vi "WCA_SET_CLNA.vi"(0 "Cartridge Band":u32=10, 1 "Slave Node in":cluster{"Address":i16, "Serial Number":i8[]}={"Address"=19, "Serial Number"=[16, 71, 55, 76, 1, 8, 0, -15]} {"Serial Number" format="%.0x"; "Address" format="%.0x"}, 2 "ObjHandle in":u32, 5 "POL":u32, 7 "sb":u32=1, 9 "CLNA_SET":T1 {"SET POL0 LNA1 STAGE3 DRAIN C" min=0 max=20 step=0.01 format="%.2f"; "SET POL0 LNA1 STAGE3 DRAIN V" min=0 max=3 step=0.01 format="%.2f"; "SET POL0 LNA1 STAGE2 DRAIN C" min=0 max=20 step=0.01 format="%.2f"; "SET POL0 LNA1 STAGE2 DRAIN V" min=0 max=3 step=0.01 format="%.2f"; "SET POL0 LNA1 STAGE1 DRAIN C" min=0 max=20 step=0.01 format="%.2f"; "SET POL0 LNA1 STAGE1 DRAIN V" min=0 max=3 step=0.01 format="%.2f"; "CLNA State" items=["Disabled", "Enabled"]}, 11 "error in (no error)":errorcluster) -> (4 "ObjHandle out":u32=92930112, 15 "error out":errorcluster)   [LabVIEW 2017]
uses:
  WCA_Global.vi
  <vilib>/express/express arith-compare/Formula/XNode/ExpressFormulaBlockNode.xnode
panel:
  # "Node Address"
  # "Serial Number"
  # "Vd [V]"
  # "Id [mA]"
  # "Stage 1"
  # "Stage 2"
  # "Stage 3"
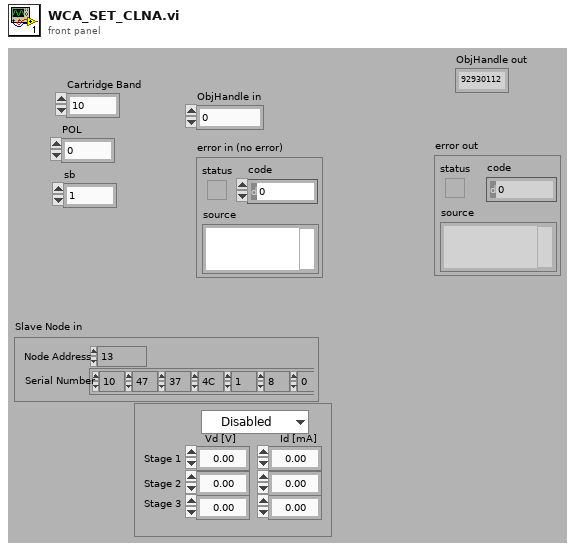
[diagram p1: front panel]
types:
  T1 = cluster{"CLNA State":u8, "SET POL0 LNA1 STAGE1 DRAIN V":sgl, "SET POL0 LNA1 STAGE1 DRAIN C":sgl, "SET POL0 LNA1 STAGE2 DRAIN V":sgl, "SET POL0 LNA1 STAGE2 DRAIN C":sgl, "SET POL0 LNA1 STAGE3 DRAIN V":sgl, "SET POL0 LNA1 STAGE3 DRAIN C":sgl}
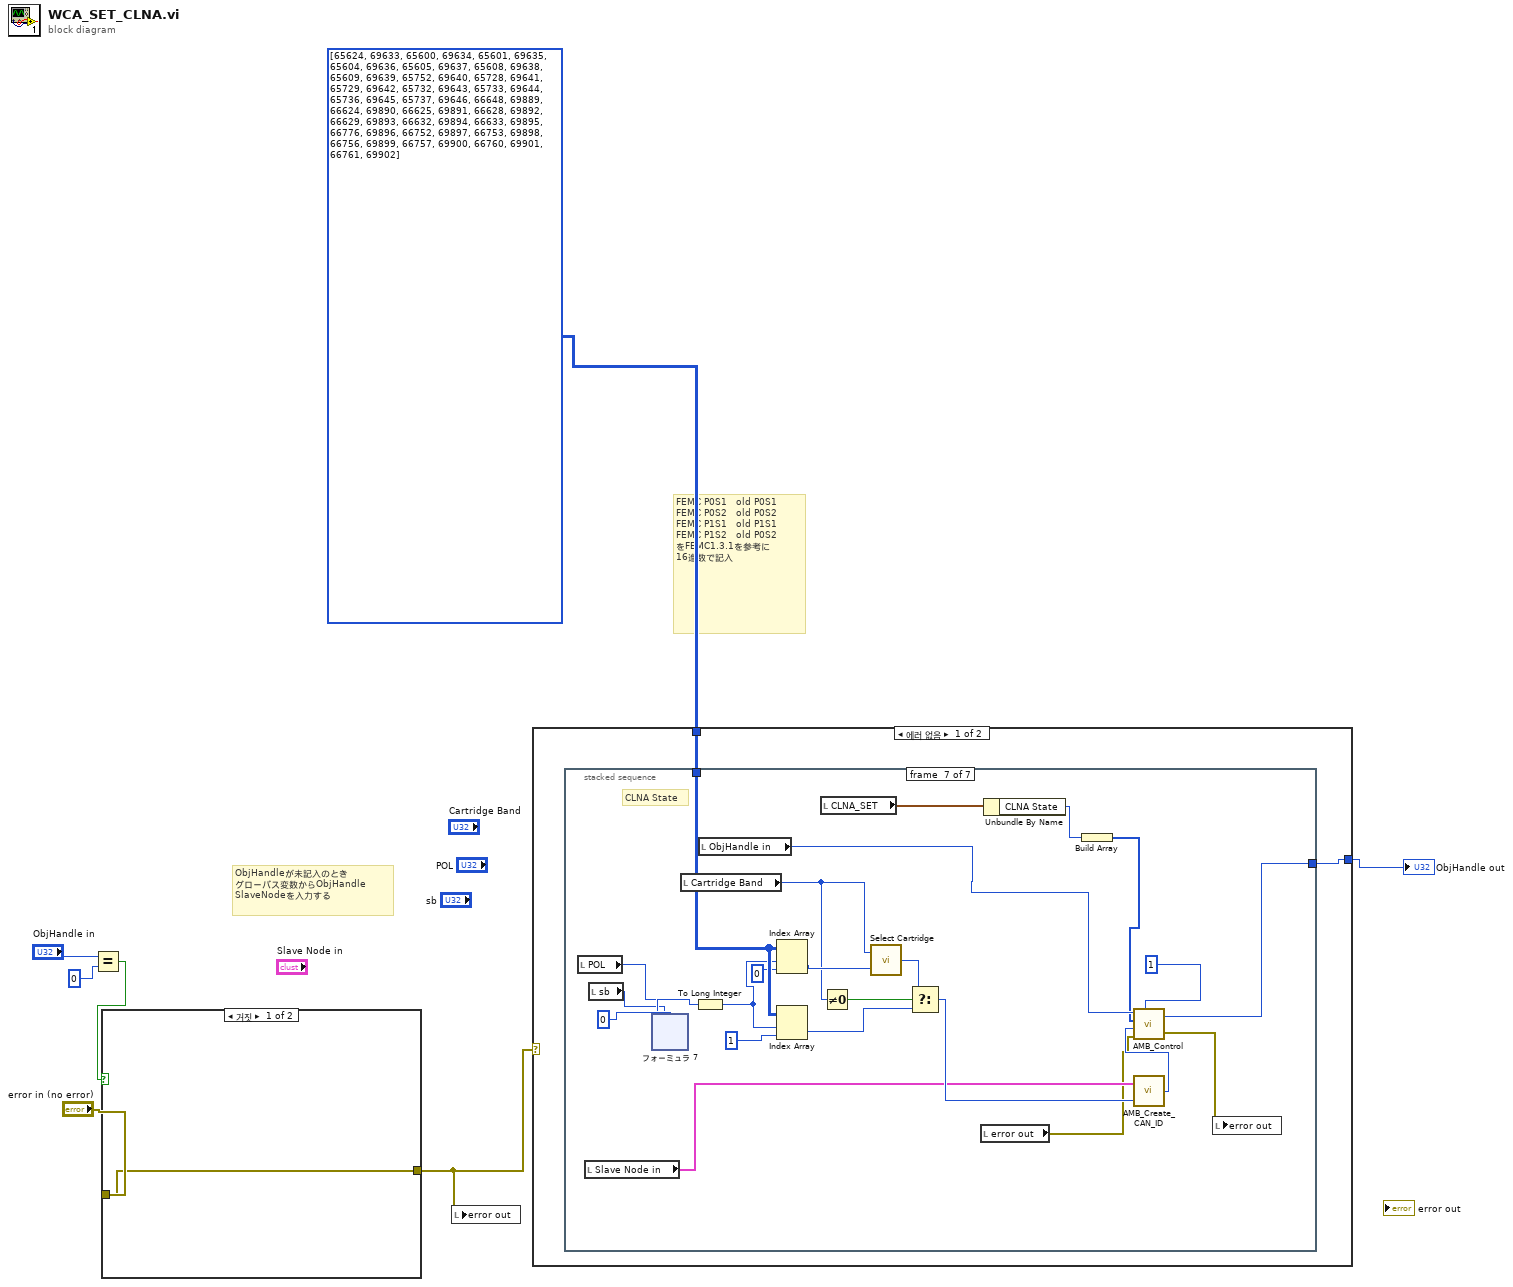
[diagram p0: block diagram]
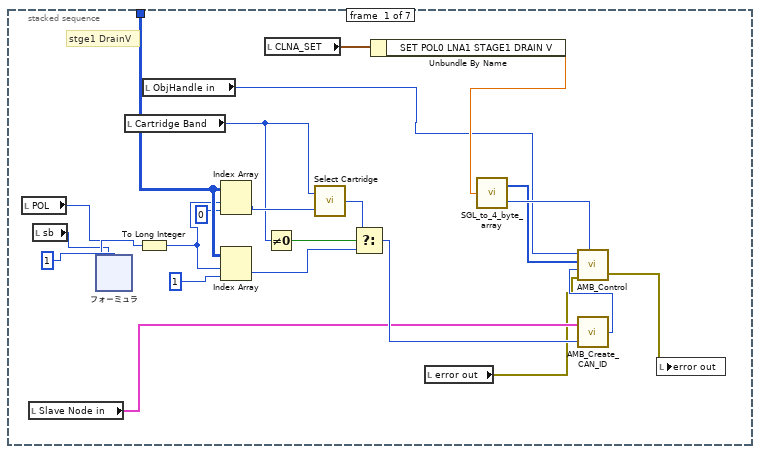
[diagram p2: hidden frame]
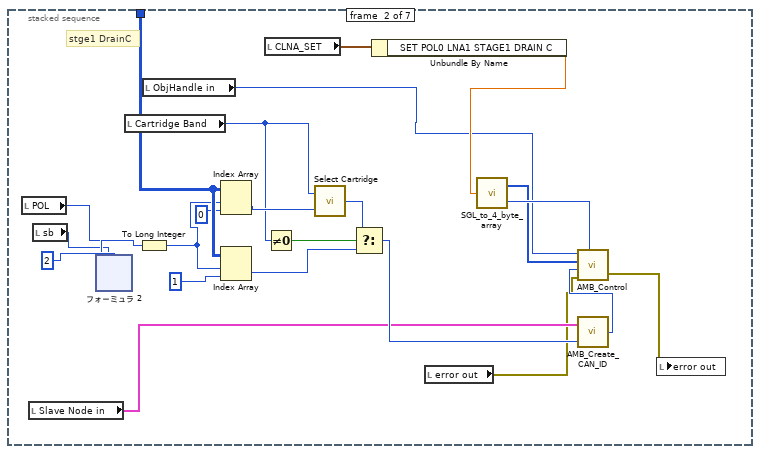
[diagram p3: hidden frame]
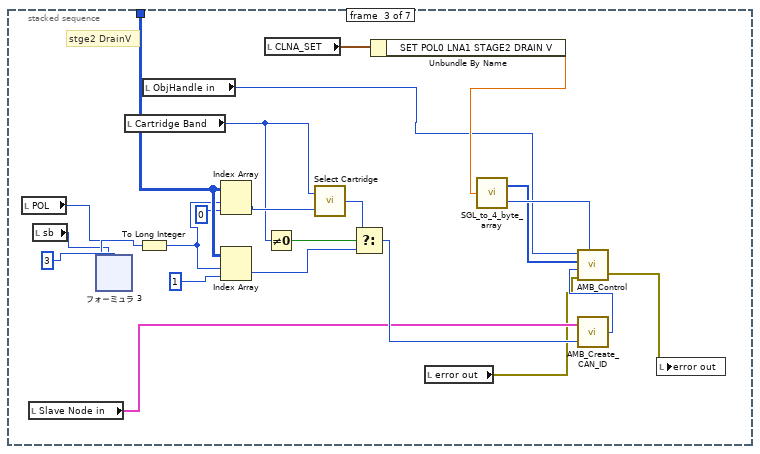
[diagram p4: hidden frame]
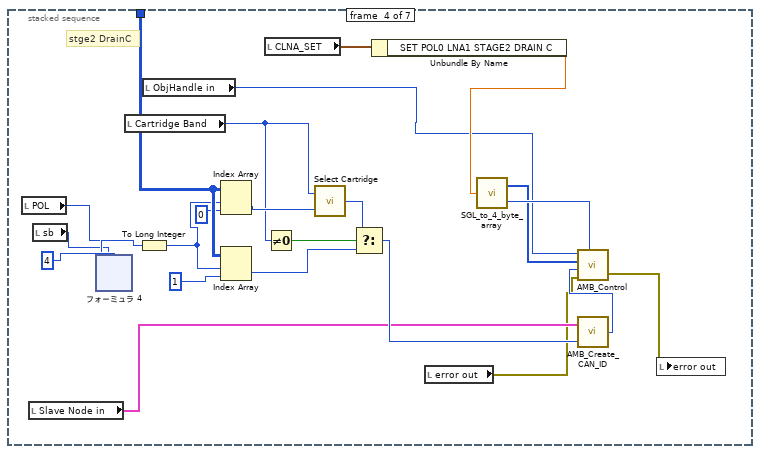
[diagram p5: hidden frame]
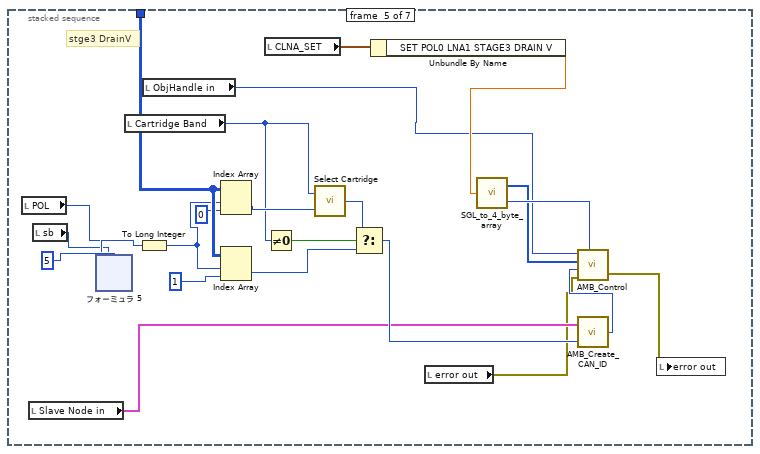
[diagram p6: hidden frame]
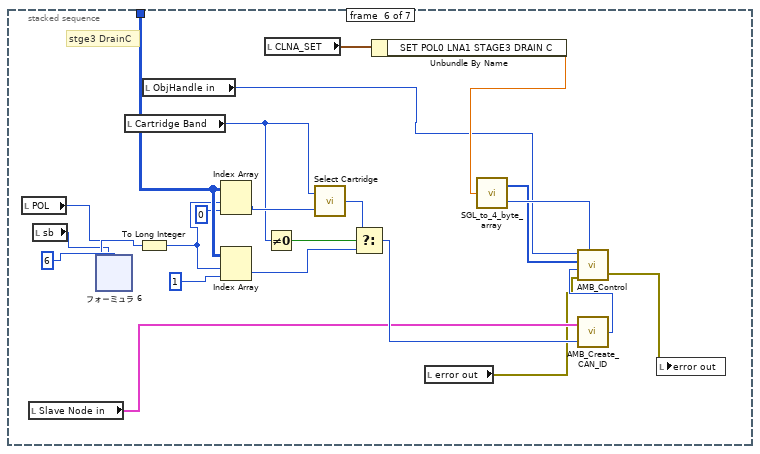
[diagram p7: hidden frame]
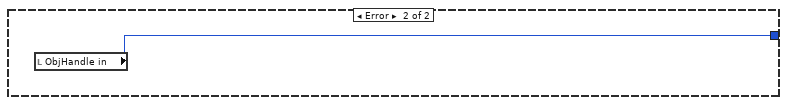
[diagram p8: hidden frame]
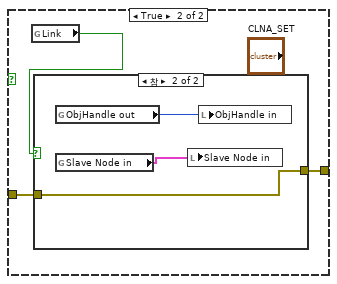
[diagram p9: hidden frame]
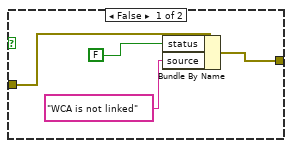
[diagram p10: hidden frame]
diagram:
  # "ObjHandleが未記入のとき\nグローバス変数からObjHandle\nSlaveNodeを入力する"
  # "FEMC P0S1   old P0S1\nFEMC P0S2   old P0S2\nFEMC P1S1   old P1S1\nFEMC P1S2   old P0S2\nをFEMC1.3.1を参考に\n16進数で記入"
  n1 = Equal?(x="ObjHandle in", y=0) -> (x = y?=w5:bool)
  n2 = case shown="거짓" w5 {
    tunnel: "error in (no error)" -> [w8 w11]
    tunnel: [w8 w10] -> w3
    frame False {
    }
    frame True {
      n3 = global read "WCA_Global.vi" "Link"() -> (w9:bool)
      n4 = case shown="참" w9 {
        tunnel: w11 -> [w15 w16]
        tunnel: [w12 w16] -> w10
        frame False {
          n5 = Bundle By Name(cluster=w15, "status"=FALSE, "source"="WCA is not linked") -> (w12:errorcluster)
        }
        frame True {
          n6 = global read "WCA_Global.vi" "ObjHandle out"() -> (w18:u32)
          n7 = global read "WCA_Global.vi" "Slave Node in"() -> (w17:cluster{"Address":i16, "Serial Number":i8[]})
          n8 = local write "Slave Node in"(w17) -> ()
          n9 = local write "ObjHandle in"(w18) -> ()
        }
      }
    }
  }
  n10 = local write "error out"(w3) -> ()
  n11 = case shown="에러 없음" w3 {
    tunnel: [w19 w267] -> w2
    tunnel: i32[][] [[65624, 69633], [65600, 69634], [65601, 69635], [65604, 69636], [65605, 69637], [65608, 69638], [65609, 69639], [65752, 69640], [65728, 69641], [65729, 69642], [65732, 69643], [65733, 69644], [65736, 69645], [65737, 69646], [66648, 69889], [66624, 69890], [66625, 69891], [66628, 69892], [66629, 69893], [66632, 69894], [66633, 69895], [66776, 69896], [66752, 69897], [66753, 69898], [66756, 69899], [66757, 69900], [66760, 69901], [66761, 69902]] -> [w20 _]
    frame No Error {
      n12 = stacked-sequence {
        tunnel: w20 -> [w43 w78 w113 w148 w183 w218 w254]
        tunnel: [_ _ _ _ _ _ w231] -> w19
        frame #0 {
          # "stge1 DrainV"
          n13 = local read "POL"() -> (w32:u32)
          n14 = local read "Slave Node in"() -> (w23:cluster{"Address":i16, "Serial Number":i8[]})
          n15 = local read "sb"() -> (w31:u32)
          n16 = xnode "フォーミュラ"("Pol"=w32, "sb"=w31, "n"=1) -> ("結果"=w35:u32)  [unwired: 1 in, 1 out]
          n17 = local read "Cartridge Band"() -> (w33:u32)
          n18 = To Long Integer(number=w35) -> (32bit integer=w34:i32)
          n19 = local read "ObjHandle in"() -> (w25:u32)
          n20 = Index Array(array=w43, index (row)=w34, index (col)=0) -> (element=w39:i32)
          n21 = Index Array(array=w43, index (row)=w34, index (col)=1) -> (element=w40:i32)
          n22 = local read "CLNA_SET"() -> (w30:T1)
          n23 = Not Equal To 0?(x=w33) -> (x != 0?=w41:bool)
          n24 = call "Select Cartridge.vi"("Relative Address in"=w39, "Cartridge band"=w33) -> ("Relative Address out"=w42:u32)
          n25 = Select(t=w42, s=w41, f=w40) -> (s? t:f=w24:u32)
          n26 = Unbundle By Name(w30) -> ("SET POL0 LNA1 STAGE1 DRAIN V"=w26:sgl)
          n27 = local read "error out"() -> (w22:errorcluster)
          n28 = call "SGL_to_4_byte_array.vi"("SGL float"=w26) -> ("SGL float encoded array of bytes"=w27:u8[], "bytes"=w28:u32)
          n29 = call "AMB_Create_CAN_ID.vi"("Relative Address in"=w24, "Slave Node in"=w23) -> ("CAN ID out"=w29:u32)
          n30 = call "AMB_Control.vi"("ObjHandle in"=w25, "Data in"=w27, "CAN ID in"=w29, "error in"=w22, "Data Length in"=w28) -> ("error out"=w21:errorcluster)  [unwired: 1 out]
          n31 = local write "error out"(w21) -> ()
        }
        frame #1 {
          # "stge1 DrainC"
          n32 = local read "POL"() -> (w67:u32)
          n33 = local read "Slave Node in"() -> (w58:cluster{"Address":i16, "Serial Number":i8[]})
          n34 = local read "sb"() -> (w66:u32)
          n35 = xnode "フォーミュラ 2"("Pol"=w67, "sb"=w66, "n"=2) -> ("結果"=w70:u32)  [unwired: 1 in, 1 out]
          n36 = local read "Cartridge Band"() -> (w68:u32)
          n37 = To Long Integer(number=w70) -> (32bit integer=w69:i32)
          n38 = local read "ObjHandle in"() -> (w60:u32)
          n39 = Index Array(array=w78, index (row)=w69, index (col)=0) -> (element=w74:i32)
          n40 = Index Array(array=w78, index (row)=w69, index (col)=1) -> (element=w75:i32)
          n41 = local read "CLNA_SET"() -> (w65:T1)
          n42 = Not Equal To 0?(x=w68) -> (x != 0?=w76:bool)
          n43 = call "Select Cartridge.vi"("Relative Address in"=w74, "Cartridge band"=w68) -> ("Relative Address out"=w77:u32)
          n44 = Select(t=w77, s=w76, f=w75) -> (s? t:f=w59:u32)
          n45 = Unbundle By Name(w65) -> ("SET POL0 LNA1 STAGE1 DRAIN C"=w61:sgl)
          n46 = local read "error out"() -> (w57:errorcluster)
          n47 = call "SGL_to_4_byte_array.vi"("SGL float"=w61) -> ("SGL float encoded array of bytes"=w62:u8[], "bytes"=w63:u32)
          n48 = call "AMB_Create_CAN_ID.vi"("Relative Address in"=w59, "Slave Node in"=w58) -> ("CAN ID out"=w64:u32)
          n49 = call "AMB_Control.vi"("ObjHandle in"=w60, "Data in"=w62, "CAN ID in"=w64, "error in"=w57, "Data Length in"=w63) -> ("error out"=w56:errorcluster)  [unwired: 1 out]
          n50 = local write "error out"(w56) -> ()
        }
        frame #2 {
          # "stge2 DrainV"
          n51 = local read "POL"() -> (w102:u32)
          n52 = local read "Slave Node in"() -> (w93:cluster{"Address":i16, "Serial Number":i8[]})
          n53 = local read "sb"() -> (w101:u32)
          n54 = xnode "フォーミュラ 3"("Pol"=w102, "sb"=w101, "n"=3) -> ("結果"=w105:u32)  [unwired: 1 in, 1 out]
          n55 = local read "Cartridge Band"() -> (w103:u32)
          n56 = To Long Integer(number=w105) -> (32bit integer=w104:i32)
          n57 = local read "ObjHandle in"() -> (w95:u32)
          n58 = Index Array(array=w113, index (row)=w104, index (col)=0) -> (element=w109:i32)
          n59 = Index Array(array=w113, index (row)=w104, index (col)=1) -> (element=w110:i32)
          n60 = local read "CLNA_SET"() -> (w100:T1)
          n61 = Not Equal To 0?(x=w103) -> (x != 0?=w111:bool)
          n62 = call "Select Cartridge.vi"("Relative Address in"=w109, "Cartridge band"=w103) -> ("Relative Address out"=w112:u32)
          n63 = Select(t=w112, s=w111, f=w110) -> (s? t:f=w94:u32)
          n64 = Unbundle By Name(w100) -> ("SET POL0 LNA1 STAGE2 DRAIN V"=w96:sgl)
          n65 = local read "error out"() -> (w92:errorcluster)
          n66 = call "SGL_to_4_byte_array.vi"("SGL float"=w96) -> ("SGL float encoded array of bytes"=w97:u8[], "bytes"=w98:u32)
          n67 = call "AMB_Create_CAN_ID.vi"("Relative Address in"=w94, "Slave Node in"=w93) -> ("CAN ID out"=w99:u32)
          n68 = call "AMB_Control.vi"("ObjHandle in"=w95, "Data in"=w97, "CAN ID in"=w99, "error in"=w92, "Data Length in"=w98) -> ("error out"=w91:errorcluster)  [unwired: 1 out]
          n69 = local write "error out"(w91) -> ()
        }
        frame #3 {
          # "stge2 DrainC"
          n70 = local read "POL"() -> (w137:u32)
          n71 = local read "Slave Node in"() -> (w128:cluster{"Address":i16, "Serial Number":i8[]})
          n72 = local read "sb"() -> (w136:u32)
          n73 = xnode "フォーミュラ 4"("Pol"=w137, "sb"=w136, "n"=4) -> ("結果"=w140:u32)  [unwired: 1 in, 1 out]
          n74 = local read "Cartridge Band"() -> (w138:u32)
          n75 = To Long Integer(number=w140) -> (32bit integer=w139:i32)
          n76 = local read "ObjHandle in"() -> (w130:u32)
          n77 = Index Array(array=w148, index (row)=w139, index (col)=0) -> (element=w144:i32)
          n78 = Index Array(array=w148, index (row)=w139, index (col)=1) -> (element=w145:i32)
          n79 = local read "CLNA_SET"() -> (w135:T1)
          n80 = Not Equal To 0?(x=w138) -> (x != 0?=w146:bool)
          n81 = call "Select Cartridge.vi"("Relative Address in"=w144, "Cartridge band"=w138) -> ("Relative Address out"=w147:u32)
          n82 = Select(t=w147, s=w146, f=w145) -> (s? t:f=w129:u32)
          n83 = Unbundle By Name(w135) -> ("SET POL0 LNA1 STAGE2 DRAIN C"=w131:sgl)
          n84 = local read "error out"() -> (w127:errorcluster)
          n85 = call "SGL_to_4_byte_array.vi"("SGL float"=w131) -> ("SGL float encoded array of bytes"=w132:u8[], "bytes"=w133:u32)
          n86 = call "AMB_Create_CAN_ID.vi"("Relative Address in"=w129, "Slave Node in"=w128) -> ("CAN ID out"=w134:u32)
          n87 = call "AMB_Control.vi"("ObjHandle in"=w130, "Data in"=w132, "CAN ID in"=w134, "error in"=w127, "Data Length in"=w133) -> ("error out"=w126:errorcluster)  [unwired: 1 out]
          n88 = local write "error out"(w126) -> ()
        }
        frame #4 {
          # "stge3 DrainV"
          n89 = local read "POL"() -> (w172:u32)
          n90 = local read "Slave Node in"() -> (w163:cluster{"Address":i16, "Serial Number":i8[]})
          n91 = local read "sb"() -> (w171:u32)
          n92 = xnode "フォーミュラ 5"("Pol"=w172, "sb"=w171, "n"=5) -> ("結果"=w175:u32)  [unwired: 1 in, 1 out]
          n93 = local read "Cartridge Band"() -> (w173:u32)
          n94 = To Long Integer(number=w175) -> (32bit integer=w174:i32)
          n95 = local read "ObjHandle in"() -> (w165:u32)
          n96 = Index Array(array=w183, index (row)=w174, index (col)=0) -> (element=w179:i32)
          n97 = Index Array(array=w183, index (row)=w174, index (col)=1) -> (element=w180:i32)
          n98 = local read "CLNA_SET"() -> (w170:T1)
          n99 = Not Equal To 0?(x=w173) -> (x != 0?=w181:bool)
          n100 = call "Select Cartridge.vi"("Relative Address in"=w179, "Cartridge band"=w173) -> ("Relative Address out"=w182:u32)
          n101 = Select(t=w182, s=w181, f=w180) -> (s? t:f=w164:u32)
          n102 = Unbundle By Name(w170) -> ("SET POL0 LNA1 STAGE3 DRAIN V"=w166:sgl)
          n103 = local read "error out"() -> (w162:errorcluster)
          n104 = call "SGL_to_4_byte_array.vi"("SGL float"=w166) -> ("SGL float encoded array of bytes"=w167:u8[], "bytes"=w168:u32)
          n105 = call "AMB_Create_CAN_ID.vi"("Relative Address in"=w164, "Slave Node in"=w163) -> ("CAN ID out"=w169:u32)
          n106 = call "AMB_Control.vi"("ObjHandle in"=w165, "Data in"=w167, "CAN ID in"=w169, "error in"=w162, "Data Length in"=w168) -> ("error out"=w161:errorcluster)  [unwired: 1 out]
          n107 = local write "error out"(w161) -> ()
        }
        frame #5 {
          # "stge3 DrainC"
          n108 = local read "POL"() -> (w207:u32)
          n109 = local read "Slave Node in"() -> (w198:cluster{"Address":i16, "Serial Number":i8[]})
          n110 = local read "sb"() -> (w206:u32)
          n111 = xnode "フォーミュラ 6"("Pol"=w207, "sb"=w206, "n"=6) -> ("結果"=w210:u32)  [unwired: 1 in, 1 out]
          n112 = local read "Cartridge Band"() -> (w208:u32)
          n113 = To Long Integer(number=w210) -> (32bit integer=w209:i32)
          n114 = local read "ObjHandle in"() -> (w200:u32)
          n115 = Index Array(array=w218, index (row)=w209, index (col)=0) -> (element=w214:i32)
          n116 = Index Array(array=w218, index (row)=w209, index (col)=1) -> (element=w215:i32)
          n117 = local read "CLNA_SET"() -> (w205:T1)
          n118 = Not Equal To 0?(x=w208) -> (x != 0?=w216:bool)
          n119 = call "Select Cartridge.vi"("Relative Address in"=w214, "Cartridge band"=w208) -> ("Relative Address out"=w217:u32)
          n120 = Select(t=w217, s=w216, f=w215) -> (s? t:f=w199:u32)
          n121 = Unbundle By Name(w205) -> ("SET POL0 LNA1 STAGE3 DRAIN C"=w201:sgl)
          n122 = local read "error out"() -> (w197:errorcluster)
          n123 = call "SGL_to_4_byte_array.vi"("SGL float"=w201) -> ("SGL float encoded array of bytes"=w202:u8[], "bytes"=w203:u32)
          n124 = call "AMB_Create_CAN_ID.vi"("Relative Address in"=w199, "Slave Node in"=w198) -> ("CAN ID out"=w204:u32)
          n125 = call "AMB_Control.vi"("ObjHandle in"=w200, "Data in"=w202, "CAN ID in"=w204, "error in"=w197, "Data Length in"=w203) -> ("error out"=w196:errorcluster)  [unwired: 1 out]
          n126 = local write "error out"(w196) -> ()
        }
        frame #6 {
          # "CLNA State"
          n127 = local read "POL"() -> (w243:u32)
          n128 = local read "Slave Node in"() -> (w237:cluster{"Address":i16, "Serial Number":i8[]})
          n129 = local read "sb"() -> (w242:u32)
          n130 = xnode "フォーミュラ 7"("Pol"=w243, "sb"=w242, "n"=0) -> ("結果"=w246:u32)  [unwired: 1 in, 1 out]
          n131 = local read "Cartridge Band"() -> (w244:u32)
          n132 = To Long Integer(number=w246) -> (32bit integer=w245:i32)
          n133 = local read "ObjHandle in"() -> (w239:u32)
          n134 = Index Array(array=w254, index (row)=w245, index (col)=0) -> (element=w250:i32)
          n135 = Index Array(array=w254, index (row)=w245, index (col)=1) -> (element=w251:i32)
          n136 = local read "CLNA_SET"() -> (w241:T1)
          n137 = Not Equal To 0?(x=w244) -> (x != 0?=w252:bool)
          n138 = call "Select Cartridge.vi"("Relative Address in"=w250, "Cartridge band"=w244) -> ("Relative Address out"=w253:u32)
          n139 = Select(t=w253, s=w252, f=w251) -> (s? t:f=w238:u32)
          n140 = local read "error out"() -> (w236:errorcluster)
          n141 = Unbundle By Name(w241) -> ("CLNA State"=w234:u8)
          n142 = Build Array(w234) -> (w233:u8[])
          n143 = call "AMB_Create_CAN_ID.vi"("Relative Address in"=w238, "Slave Node in"=w237) -> ("CAN ID out"=w240:u32)
          n144 = call "AMB_Control.vi"("ObjHandle in"=w239, "Data in"=w233, "CAN ID in"=w240, "error in"=w236, "Data Length in"=1) -> ("ObjHandle out"=w231:u32, "error out"=w235:errorcluster)
          n145 = local write "error out"(w235) -> ()
        }
      }
    }
    frame Error {
      n146 = local read "ObjHandle in"() -> (w267:u32)
    }
  }
  "ObjHandle out" <- w2
